vi "LoadFileData.vi"(8 "error in (no error)":errorcluster, 10 "NameFiles":string, 11 "ClassDataTree in":refnum<class "ClassDataTree.lvclass">) -> (0 "error out":errorcluster, 3 "ClassDataTree out":refnum<class "ClassDataTree.lvclass">)   [LabVIEW 2010, in "ClassDataTree.lvclass"]
uses:
  ClassDataTree.lvclass
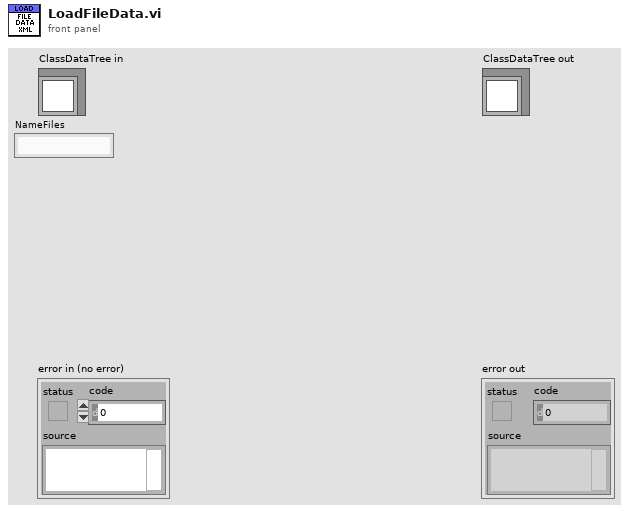
[diagram p1: front panel]
types:
  T1 = cluster{"Get Parent":string, "Active Item Tag":string, "Cell String":string, "Indent Level":i32}[]
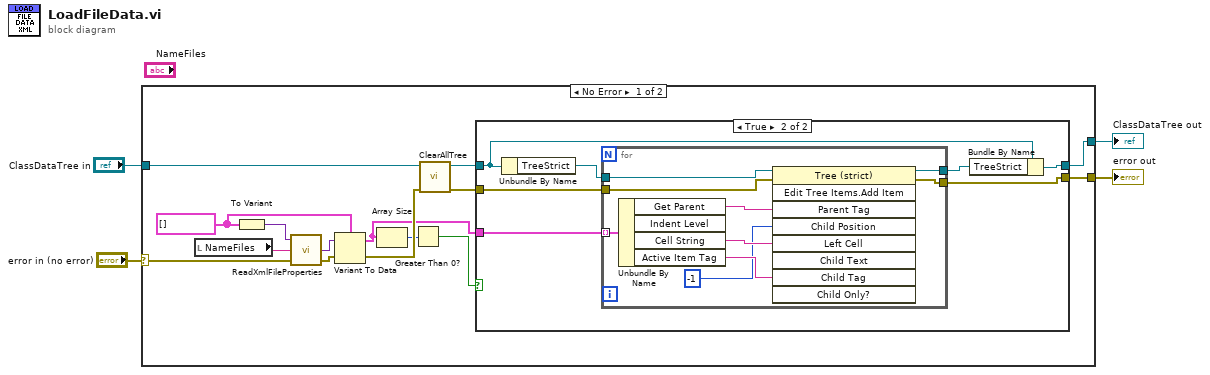
[diagram p0: block diagram]
diagram:
  n1 = case shown="No Error" "error in (no error)" {
    selector: "error in (no error)" -> [w13 w39]
    tunnel: [w15 w39] -> w3
    tunnel: [w5 w38] -> w1
    tunnel: "ClassDataTree in" -> [w10 w38]
    frame No Error {
      w14 = T1 []
      n2 = local read "NameFiles"() -> (w19:string)
      n3 = To Variant(anything=w14) -> (Variant=w18:variant)
      n4 = call "ReadXmlFileProperties.vi"("error in"=w13, "NameFileAndType"=w19, "parameters"=w18) -> ("error out"=w16:errorcluster, "OutputParamReadFile"=w17:variant)  [unwired: 1 out]
      n5 = Variant To Data(error in=w16, Variant=w17, type=w14) -> (error out=w12:errorcluster, data=w9:cluster{})
      n6 = Array Size(array=w9) -> (size(s)=w8:i32)
      n7 = Greater Than 0?(x=w8) -> (x > 0?=w7:bool)
      n8 = call-dynamic "ClearAllTree.vi"("error in (no error)"=w12, "ClassDataTree in"=w10) -> ("error out"=w11:errorcluster, "ClassDataTree out"=w6:refnum<class "ClassDataTree.lvclass">)  [unwired: 8 in]
      n9 = case shown="True" w7 {
        tunnel: [w21 w28] -> w15
        tunnel: w9 -> [_ w22]
        tunnel: w11 -> [w21 w27]
        tunnel: w6 -> [w20 w23]
        tunnel: [w20 w24] -> w5
        frame False {
        }
        frame True {
          n10 = Unbundle By Name(w23) -> ("TreeStrict"=w26:refnum<vi>)
          n11 = for {
            tunnel: w27 -> [w37]
            tunnel: [w35] -> w28
            tunnel: [w36] -> w25
            tunnel: w26 -> [w31]
            tunnel: w22 -> [w29] mode=indexing
            n12 = Unbundle By Name(w29) -> ("Get Parent"=w34:string, "Cell String"=w33:string, "Active Item Tag"=w32:string)  [unwired: 1 out]
            n13 = invoke class="Tree (strict)" method="Edit Tree Items.Add Item"(reference=w31, error in=w37, "Parent Tag"=w34, "Child Position"=-1, "Left Cell"=w33, "Child Tag"=w32) -> (reference out=w36:refnum<vi>, error out=w35:errorcluster)  [unwired: 3 in, 7 out]
          }
          n14 = Bundle By Name(cluster=w23, "TreeStrict"=w25) -> (w24:refnum<class "ClassDataTree.lvclass">)
        }
      }
    }
    frame Error {
    }
  }
  "error out" <- w3
  "ClassDataTree out" <- w1
